vi "Get Model Parameters From File.vi"(8 "error in (no error)":errorcluster, 10 "Base Path For Model":path=path "D:/Dropbox/Matlab/Hellicopter") -> (0 "error out":errorcluster, 2 "Model Parameters":T4 {"DT KF State-Space Model"."Transport Delay" format="%.2f"; "DT KF State-Space Model"."D" format="%#.2g"; "DT KF State-Space Model"."C" format="%#.2g"; "DT KF State-Space Model"."B" format="%#.2g"; "DT KF State-Space Model"."A" format="%#.2g"; "DT KF State-Space Model"."properties"."Sampling Time" format="%#.6p"; "DT KF State-Space Model"."properties"."Output Delays" format="%.4f"; "DT KF State-Space Model"."properties"."Input Delays" format="%.4f"})   [LabVIEW 2017]
uses:
  <vilib>/Analysis/Matrix/Datatypes/RealMatrix.ctl
  <vilib>/addons/Control Design/_Model Construction/Model Typedefs.llb/CD State Space Model (MIMO).ctl
  <vilib>/addons/Control Design/_Model Construction/Model Typedefs.llb/CD General Elements.ctl
  <vilib>/Utility/file.llb/Read Delimited Spreadsheet (DBL).vi
  <vilib>/addons/Control Design/_Model Construction/Model Creation.llb/Model Creation SubVI/cd_Create State Space Model.vi
  <vilib>/addons/Control Design/_Model Construction/Model Information.llb/Model Information SubVIs/cd_Set Names To SS Model.vi
  <vilib>/Analysis/Matrix/Numeric/Conversions/Array To Matrix - RA2.vi
  <vilib>/addons/Control Design/_Model Construction/NI_LinSys_Model Creation.lvlib
  <vilib>/addons/Control Design/_Model Construction/NI_LinSys_Model Information.lvlib
  <vilib>/Analysis/Matrix/NI_Matrix.lvlib
  <vilib>/addons/Control Design/_Model Construction/NI_LinSys_Model Typedefs.lvlib
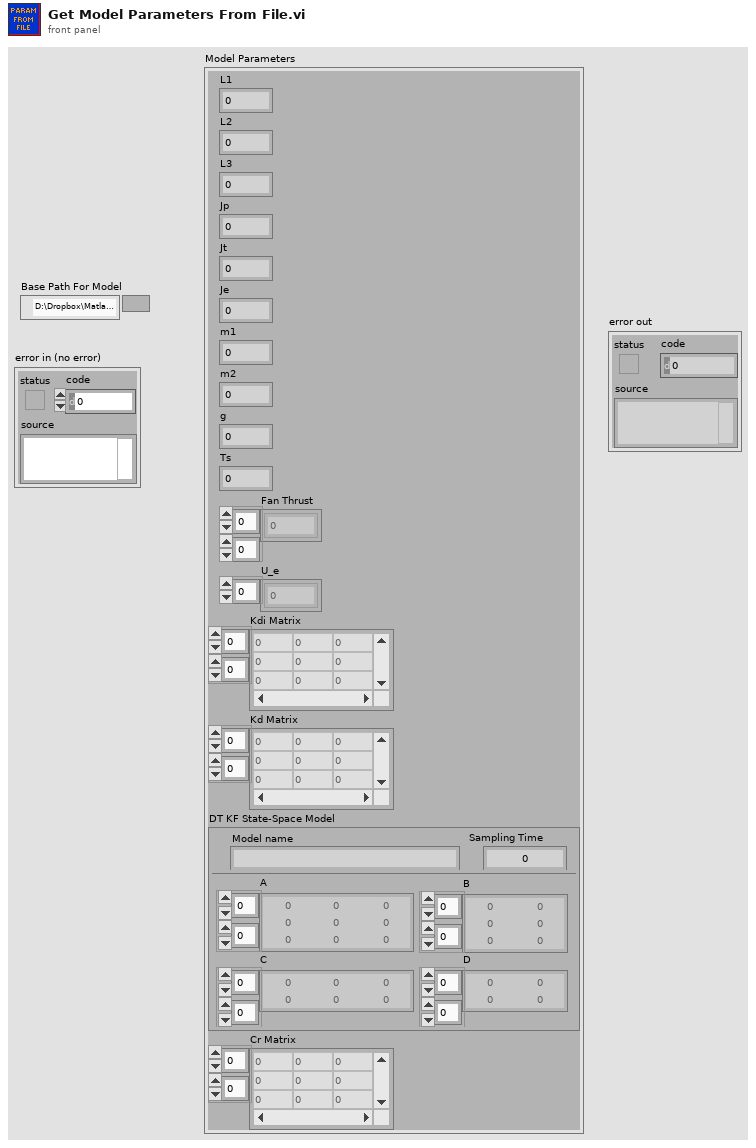
[diagram p1: front panel]
types:
  T1 = typedef "NI_Matrix.lvlib/RealMatrix.ctl" = dbl[][]
  T2 = typedef "NI_LinSys_Model Typedefs.lvlib/CD State Space Model (MIMO).ctl" = cluster{"properties":T3, "A":dbl[][], "B":dbl[][], "C":dbl[][], "D":dbl[][], "StateNames":string[], "Transport Delay":dbl[][]}
  T3 = typedef "NI_LinSys_Model Typedefs.lvlib/CD General Elements.ctl" = cluster{"Model name":string, "Input names":string[], "Output names":string[], "Input Delays":dbl[], "Output Delays":dbl[], "Sampling Time":dbl, "Notes":string}
  T4 = cluster{"L1":dbl, "L2":dbl, "L3":dbl, "Jp":dbl, "Jt":dbl, "Je":dbl, "m1":dbl, "m2":dbl, "g":dbl, "Ts":dbl, "Fan Thrust":dbl[][], "U_e":dbl[], "Kdi Matrix":T1, "Kd Matrix":T1, "DT KF State-Space Model":T2, "Cr Matrix":T1}
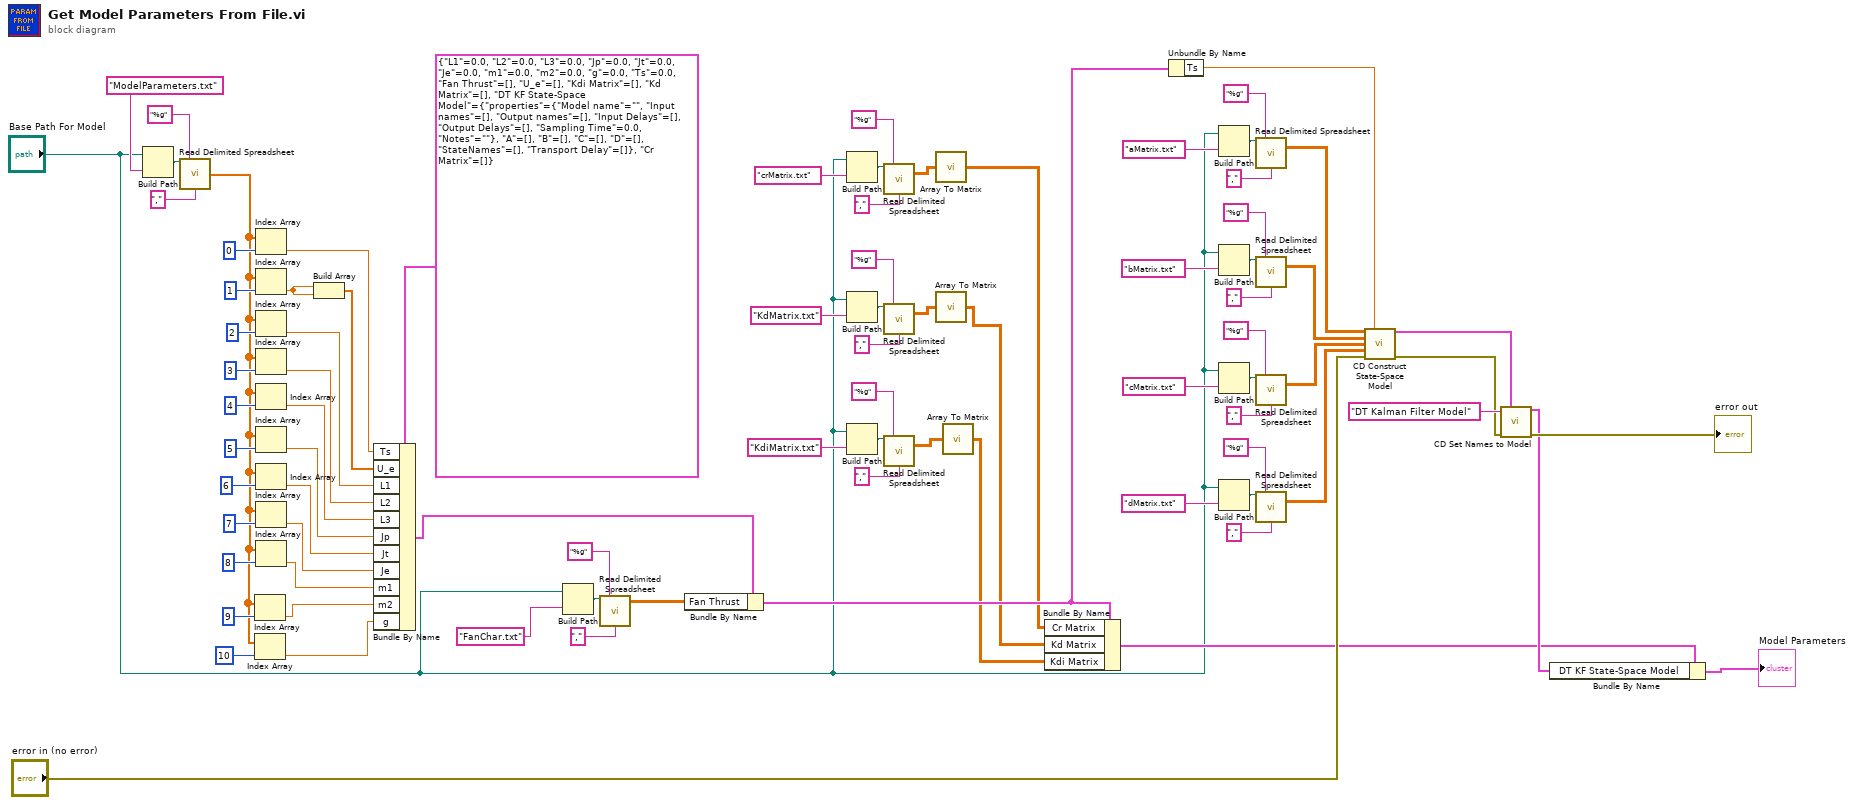
[diagram p0: block diagram]
diagram:
  n1 = Build Path(base path="Base Path For Model", name or relative path="ModelParameters.txt") -> (appended path=w82:path)
  n2 = call-poly <vilib>:"Read Delimited Spreadsheet.vi"("file path (dialog if empty)"=w82, "format (%.3f)"="%g", "delimiter (\\t)"="," ("delimiter (\\t)")) -> ("first row"=w60:dbl[])  [unwired: 7 in, 5 out]
  n3 = Index Array(array=w60, index=9) -> (element=w59:dbl)
  n4 = Index Array(array=w60, index=10) -> (element=w58:dbl)
  n5 = Index Array(array=w60, index=0) -> (element=w70:dbl)
  n6 = Index Array(array=w60, index=1) -> (element=w16:dbl)
  n7 = Index Array(array=w60, index=2) -> (element=w69:dbl)
  n8 = Index Array(array=w60, index=3) -> (element=w68:dbl)
  n9 = Index Array(array=w60, index=4) -> (element=w67:dbl)
  n10 = Index Array(array=w60, index=5) -> (element=w66:dbl)
  n11 = Index Array(array=w60, index=6) -> (element=w65:dbl)
  n12 = Index Array(array=w60, index=7) -> (element=w64:dbl)
  n13 = Index Array(array=w60, index=8) -> (element=w63:dbl)
  n14 = Build Array(w16, w16) -> (w15:dbl[])
  n15 = Bundle By Name(cluster=T4 {"L1"=0.0, "L2"=0.0, "L3"=0.0, "Jp"=0.0, "Jt"=0.0, "Je"=0.0, "m1"=0.0, "m2"=0.0, "g"=0.0, "Ts"=0.0, "Fan Thrust"=[], "U_e"=[], "Kdi Matrix"=[], "Kd Matrix"=[], "DT KF State-Space Model"={"properties"={"Model name"="", "Input names"=[], "Output names"=[], "Input Delays"=[], "Output Delays"=[], "Sampling Time"=0.0, "Notes"=""}, "A"=[], "B"=[], "C"=[], "D"=[], "StateNames"=[], "Transport Delay"=[]}, "Cr Matrix"=[]}, "Ts"=w70, "U_e"=w15, "L1"=w69, "L2"=w68, "L3"=w67, "Jp"=w66, "Jt"=w65, "Je"=w64, "m1"=w63, "m2"=w59, "g"=w58) -> (w53:T4)
  n16 = Build Path(base path="Base Path For Model", name or relative path="FanChar.txt") -> (appended path=w55:path)
  n17 = call-poly <vilib>:"Read Delimited Spreadsheet.vi"("file path (dialog if empty)"=w55, "format (%.3f)"="%g", "delimiter (\\t)"="," ("delimiter (\\t)")) -> ("all rows"=w52:dbl[][])  [unwired: 7 in, 5 out]
  n18 = Bundle By Name(cluster=w53, "Fan Thrust"=w52) -> (w14:T4)
  n19 = Build Path(base path="Base Path For Model", name or relative path="crMatrix.txt") -> (appended path=w8:path)
  n20 = Build Path(base path="Base Path For Model", name or relative path="KdMatrix.txt") -> (appended path=w20:path)
  n21 = Build Path(base path="Base Path For Model", name or relative path="KdiMatrix.txt") -> (appended path=w25:path)
  n22 = call-poly <vilib>:"Read Delimited Spreadsheet.vi"("file path (dialog if empty)"=w8, "format (%.3f)"="%g", "delimiter (\\t)"="," ("delimiter (\\t)")) -> ("all rows"=w10:dbl[][])  [unwired: 7 in, 5 out]
  n23 = call-poly <vilib>:"Read Delimited Spreadsheet.vi"("file path (dialog if empty)"=w20, "format (%.3f)"="%g", "delimiter (\\t)"="," ("delimiter (\\t)")) -> ("all rows"=w18:dbl[][])  [unwired: 7 in, 5 out]
  n24 = call-poly <vilib>:"Read Delimited Spreadsheet.vi"("file path (dialog if empty)"=w25, "format (%.3f)"="%g", "delimiter (\\t)"="," ("delimiter (\\t)")) -> ("all rows"=w17:dbl[][])  [unwired: 7 in, 5 out]
  n25 = call-poly <vilib>:"Array To Matrix.vi"("Real 2D Array"=w10) -> ("Real Matrix"=w2:T1)
  n26 = call-poly <vilib>:"Array To Matrix.vi"("Real 2D Array"=w18) -> ("Real Matrix"=w3:T1)
  n27 = call-poly <vilib>:"Array To Matrix.vi"("Real 2D Array"=w17) -> ("Real Matrix"=w4:T1)
  n28 = Bundle By Name(cluster=w14, "Cr Matrix"=w2, "Kd Matrix"=w3, "Kdi Matrix"=w4) -> (w11:T4)
  n29 = Unbundle By Name(w14) -> ("Ts"=w13:dbl)
  n30 = Build Path(base path="Base Path For Model", name or relative path="aMatrix.txt") -> (appended path=w50:path)
  n31 = Build Path(base path="Base Path For Model", name or relative path="bMatrix.txt") -> (appended path=w45:path)
  n32 = Build Path(base path="Base Path For Model", name or relative path="cMatrix.txt") -> (appended path=w42:path)
  n33 = Build Path(base path="Base Path For Model", name or relative path="dMatrix.txt") -> (appended path=w37:path)
  n34 = call-poly <vilib>:"Read Delimited Spreadsheet.vi"("file path (dialog if empty)"=w50, "format (%.3f)"="%g", "delimiter (\\t)"="," ("delimiter (\\t)")) -> ("all rows"=w35:dbl[][])  [unwired: 7 in, 5 out]
  n35 = call-poly <vilib>:"Read Delimited Spreadsheet.vi"("file path (dialog if empty)"=w45, "format (%.3f)"="%g", "delimiter (\\t)"="," ("delimiter (\\t)")) -> ("all rows"=w34:dbl[][])  [unwired: 7 in, 5 out]
  n36 = call-poly <vilib>:"Read Delimited Spreadsheet.vi"("file path (dialog if empty)"=w42, "format (%.3f)"="%g", "delimiter (\\t)"="," ("delimiter (\\t)")) -> ("all rows"=w33:dbl[][])  [unwired: 7 in, 5 out]
  n37 = call-poly <vilib>:"Read Delimited Spreadsheet.vi"("file path (dialog if empty)"=w37, "format (%.3f)"="%g", "delimiter (\\t)"="," ("delimiter (\\t)")) -> ("all rows"=w32:dbl[][])  [unwired: 7 in, 5 out]
  n38 = call-poly <vilib>:"CD Construct State-Space Model.vi"("A"=w35, "Sampling Time (s)"=w13, "B"=w34, "C"=w33, "D"=w32, "error in (no error)"="error in (no error)") -> ("State-Space Model"=w31:T2, "error out"=w28:errorcluster)  [unwired: 8 in]
  n39 = call-poly <vilib>:"CD Set Names to Model.vi"("Model Name"="DT Kalman Filter Model", "State-Space Model In"=w31, "error in (no error)"=w28) -> ("Model Out"=w12:T2, "error out"=→"error out":errorcluster)  [unwired: 11 in]
  n40 = Bundle By Name(cluster=w11, "DT KF State-Space Model"=w12) -> (→"Model Parameters":T4)
